vi "PenaltyAttackerRole.vi"(8 "error in (no error)":errorcluster, 10 "Game in":refnum<class "Game.lvclass">, 11 "PenaltyAttackerRole in":refnum<class "PenaltyAttackerRole.lvclass">) -> (0 "error out":errorcluster, 2 "Robot out":refnum<class "Robot.lvclass">, 3 "PenaltyAttackerRole out":refnum<class "PenaltyAttackerRole.lvclass">)   [LabVIEW 2023, in "PenaltyAttackerRole.lvclass"]
uses:
  PenaltyAttackerRole.lvclass
  Robot_class/Robot.lvclass
  Game_class/Game.lvclass
  Role_class/Role.lvclass/Role.ctl
  Tacticbook_class/Tacticbook.lvclass/Tacticbook.ctl
  Tacticbook_class/Read ShootTactic.vi
  ShootTactic_class/Read States.vi
  Tacticbook_class/Write ShootTactic.vi
  Role_class/Read Tacticbook.vi
  Role_class/Read tactic_index.vi
  Role_class/Write Tacticbook.vi
  Role_class/Write tactic_index.vi
  Role_class/Read RobotRef.vi
  Tacticbook_class/Tacticbook.lvclass
  ShootTactic_class/ShootTactic.lvclass
panel:
  out "Game out":refnum<class "Game.lvclass">
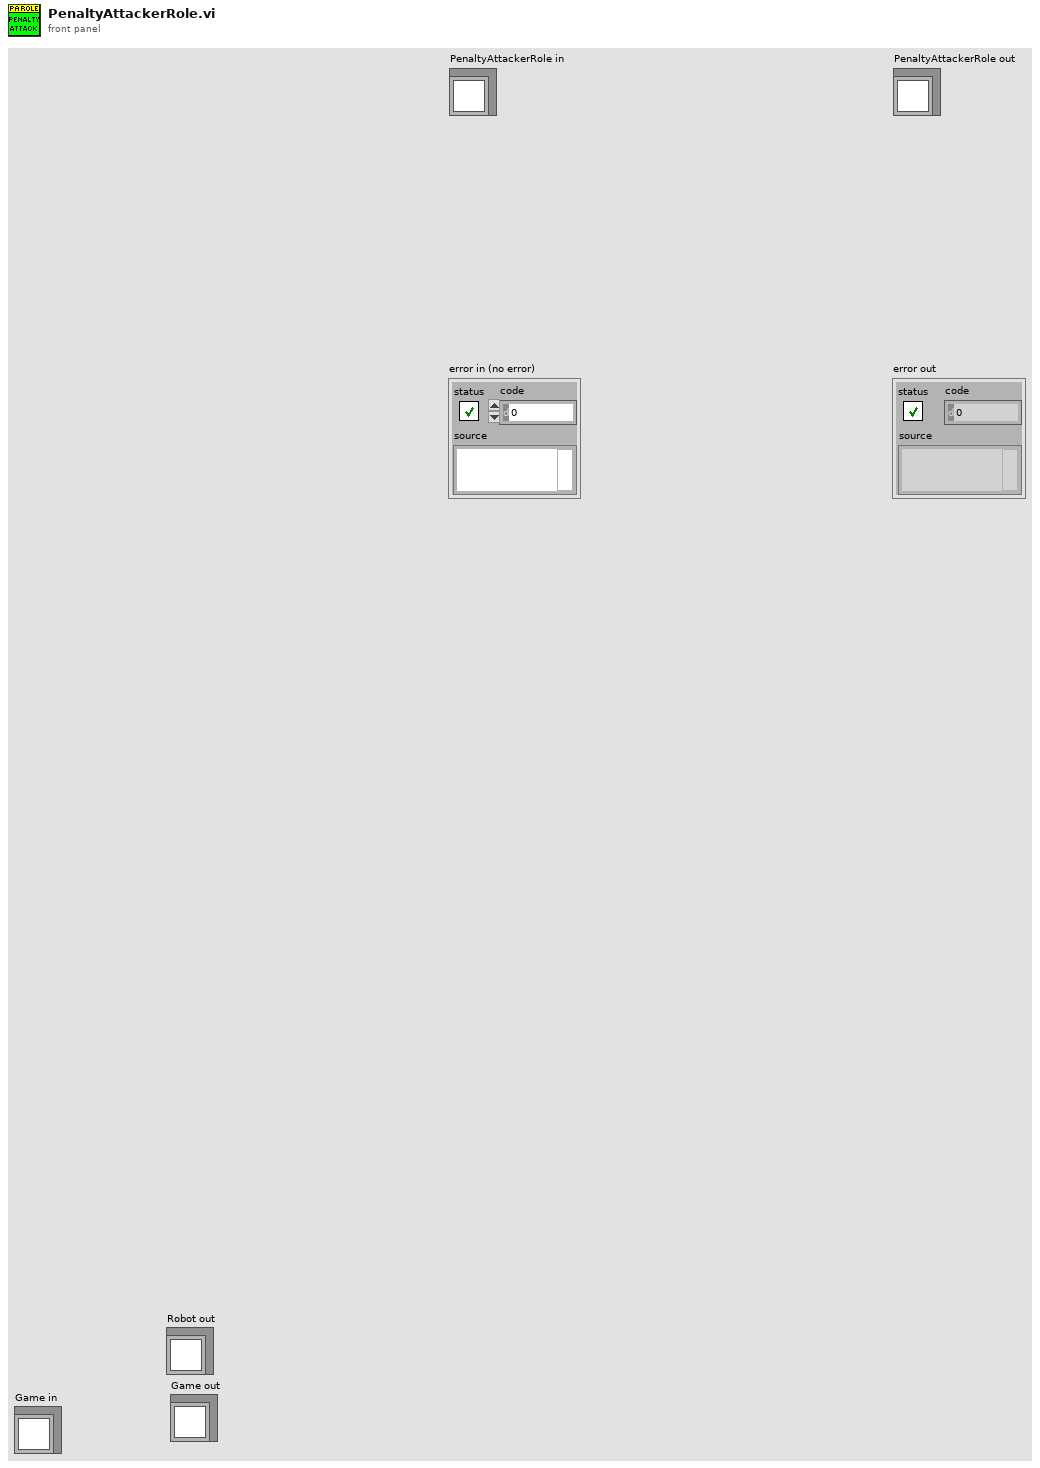
[diagram p1: front panel]
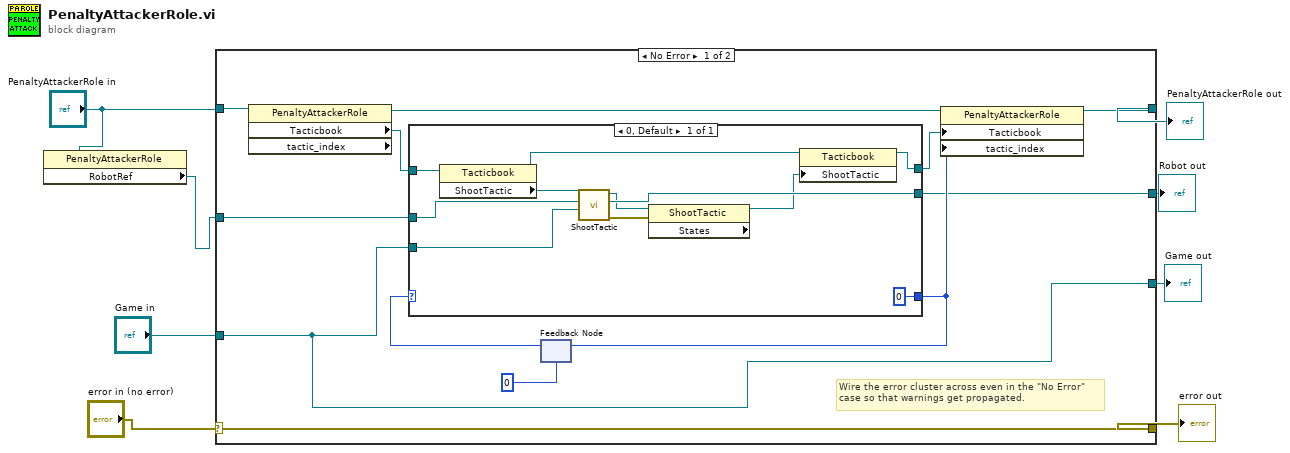
[diagram p0: block diagram]
diagram:
  n1 = property class="PenaltyAttackerRole"(reference="PenaltyAttackerRole in") -> ("RobotRef"=w1:refnum<class "Robot.lvclass">)  [unwired: 1 in, 2 out]
  n2 = case shown="No Error" "error in (no error)" {
    selector: "error in (no error)" -> [w20 w35]
    tunnel: [w20 w35] -> w3
    tunnel: [w18 w34] -> w5
    tunnel: "PenaltyAttackerRole in" -> [w19 w34]
    tunnel: w1 -> [w12 w33]
    tunnel: [w11 w33] -> w8
    tunnel: [w9 w32] -> w7
    tunnel: "Game in" -> [w9 w32]
    frame No Error {
      # "Wire the error cluster across even in the \"No Error\"\ncase so that warnings get propagated."
      n3 = property class="PenaltyAttackerRole" props=["Tacticbook", "tactic_index"](reference=w19) -> (reference out=w17:refnum<class "PenaltyAttackerRole.lvclass">, "Tacticbook"=w14:refnum<class "Tacticbook.lvclass">)  [unwired: 1 in, 2 out]
      n4 = feedback #1(0) -> (w15:i32)
      n5 = case shown="0, Default" w15 {
        tunnel: [0] -> w13
        tunnel: w14 -> [w31]
        tunnel: w12 -> [w24]
        tunnel: [w30] -> w11
        tunnel: [w26] -> w10
        tunnel: w9 -> [w22]
        frame 0, Default {
          n6 = property class="Tacticbook"(reference=w31) -> (reference out=w28:refnum<class "Tacticbook.lvclass">, "ShootTactic"=w25:refnum<class "ShootTactic.lvclass">)  [unwired: 1 in, 1 out]
          n7 = call "ShootTactic.vi"("Game in"=w22, "Robot"=w24, "ShootTactic in"=w25) -> ("error out"=w29:errorcluster, "Robot out"=w30:refnum<class "Robot.lvclass">, "ShootTactic out"=w23:refnum<class "ShootTactic.lvclass">)  [unwired: 6 in]
          n8 = property class="ShootTactic" props=["States"](reference=w23, error in=w29) -> (reference out=w27:refnum<class "ShootTactic.lvclass">)  [unwired: 2 out]
          n9 = property class="Tacticbook"(reference=w28, "ShootTactic"=w27) -> (reference out=w26:refnum<class "Tacticbook.lvclass">)  [unwired: 1 in, 1 out]
        }
      }
      n10 = feedback-in #1(w13) -> ()
      n11 = property class="PenaltyAttackerRole"(reference=w17, "Tacticbook"=w10, "tactic_index"=w13) -> (reference out=w18:refnum<class "PenaltyAttackerRole.lvclass">)  [unwired: 1 in, 1 out]
    }
    frame Error {
    }
  }
  "error out" <- w3
  "PenaltyAttackerRole out" <- w5
  "Robot out" <- w8
  "Game out" <- w7
